vi "AnalogInput_PanelSim_Global.vi"(0 "menu":T5=enum."set avg_bits", 5 "Channel":T4, 9 "Value Set":dbl format="%#.4f", 11 "error in (no error)":errorcluster, 12 "String Value":string) -> (10 "AI Value out":T1={"type"="AI", "device"="", "name"="", "data"={"<init"=FALSE, "<avg_bits"=0, "<oversample_bits"=0, ">voltage"=0.0, " Accum Object"={"<init"=FALSE, ">value"=0.0, ">count"=0, "<center"=0, "<deadband"=0}}}, 15 "error out":errorcluster)   [LabVIEW 2019]
doc: "This is used to set and get the last motor output values. This is needed for simulation, since we cannot read these values from the hardware.\n\nThis software is licensed. Open the labview\\readme\\WPI Robotics Library Open Source License.txt file for more information."
uses:
  AI Accum proto.ctl
  AI Data proto.ctl
  AI proto.ctl
  <vilib>/Rock Robotics/SystemInterfaces/AI/FPGA_AIChannel.ctl
  AI Update Ops.ctl
panel:
  out "All Values":T1[](array[typedef])
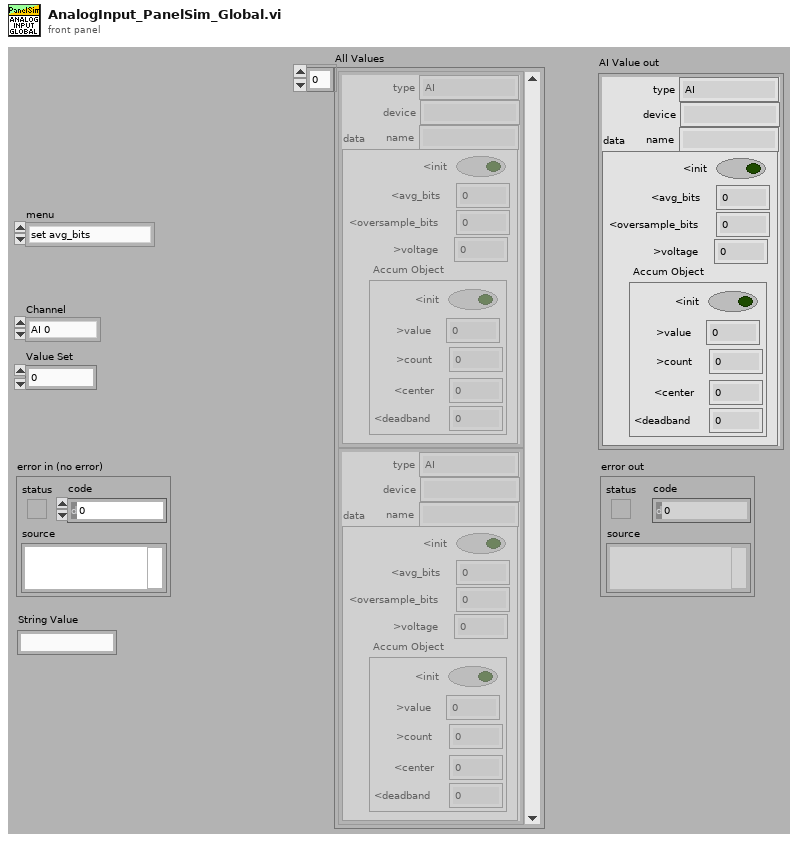
[diagram p1: front panel]
types:
  T1 = typedef "AI proto.ctl" = cluster{"type":string, "device":string, "name":string, "data":T2}
  T2 = typedef "AI Data proto.ctl" = cluster{"<init":bool, "<avg_bits":i32, "<oversample_bits":i32, ">voltage":dbl, " Accum Object":T3}
  T3 = typedef "AI Accum proto.ctl" = cluster{"<init":bool, ">value":dbl, ">count":i32, "<center":i32, "<deadband":i32}
  T4 = typedef "FPGA_AIChannel.ctl" = enum8{"AI 0", "AI 1", "AI 2", "AI 3", "AI MXP 0", "AI MXP 1", "AI MXP 2", "AI MXP 3", "Invalid"}
  T5 = typedef "AI Update Ops.ctl" = enum16{"set init", "set avg_bits", "set oversample_bits", "set voltage", "set Accum_init", "set Accum_value", "set Accum_count", "set Accum_center", "set Accum_deadband", "get", "delete", "JSON update", "set  name", "transmit initial", "reset"}
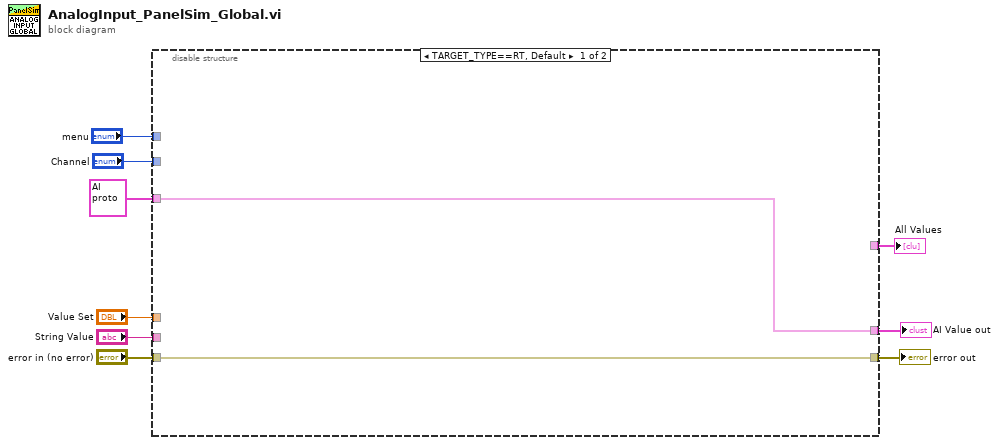
[diagram p0: block diagram]
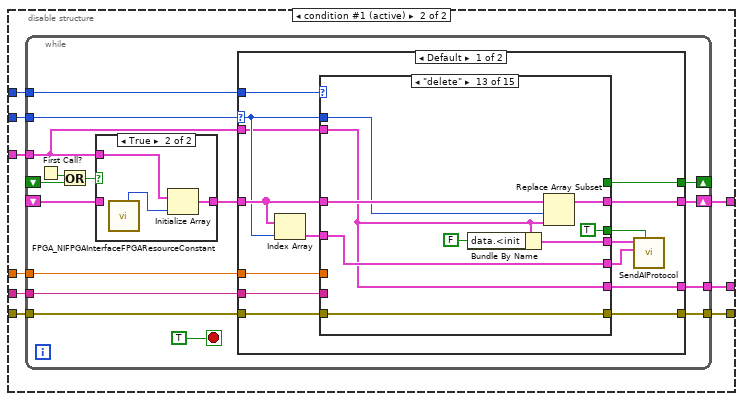
[diagram p2: hidden frame]
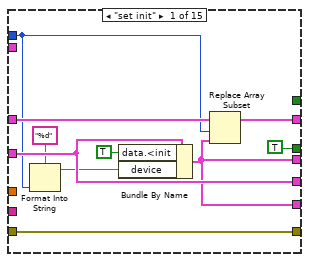
[diagram p3: hidden frame]
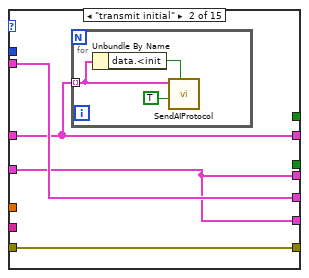
[diagram p4: hidden frame]
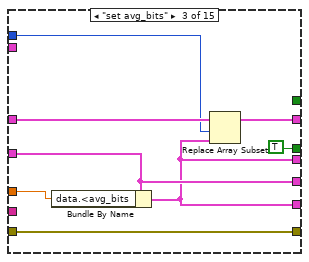
[diagram p5: hidden frame]
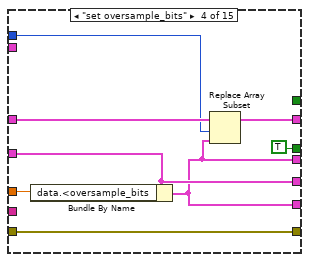
[diagram p6: hidden frame]
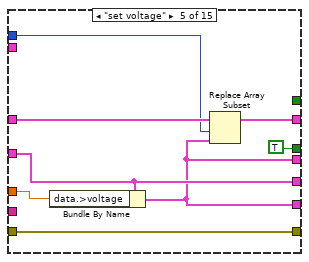
[diagram p7: hidden frame]
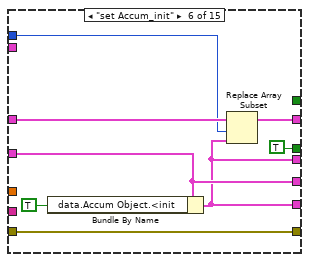
[diagram p8: hidden frame]
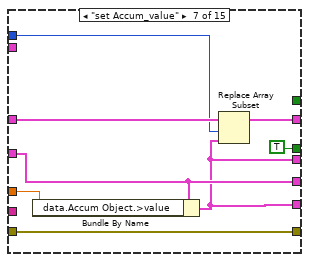
[diagram p9: hidden frame]
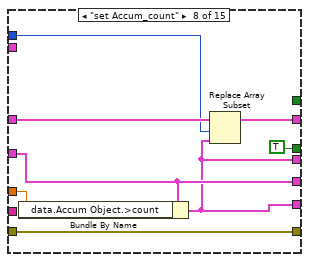
[diagram p10: hidden frame]
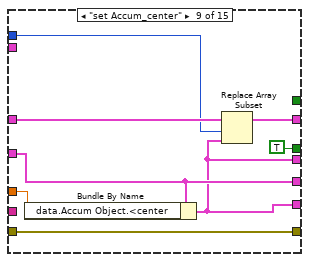
[diagram p11: hidden frame]
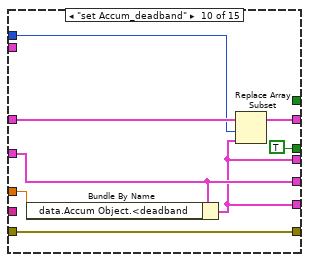
[diagram p12: hidden frame]
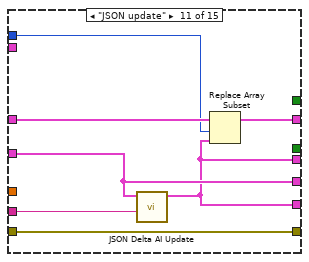
[diagram p13: hidden frame]
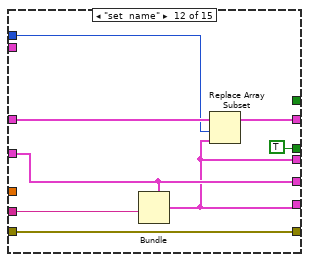
[diagram p14: hidden frame]
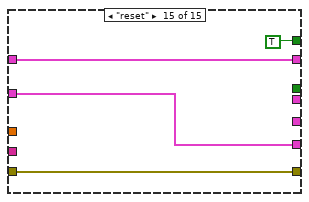
[diagram p16: hidden frame]
diagram:
  n1 = disable-structure shown="TARGET_TYPE==RT, Default" {
    disable-tunnel: "menu" -> [_ w20]
    disable-tunnel: [w11 w19] -> w8
    disable-tunnel: "error in (no error)" -> [w11 w18]
    disable-tunnel: [_ w17] -> w6
    disable-tunnel: "Value Set" -> [_ w16]
    disable-tunnel: "Channel" -> [_ w15]
    disable-tunnel: [w10 w14] -> w1
    disable-tunnel: T1 {"type"="AI", "device"="", "name"="", "data"={"<init"=FALSE, "<avg_bits"=0, "<oversample_bits"=0, ">voltage"=0.0, " Accum Object"={"<init"=FALSE, ">value"=0.0, ">count"=0, "<center"=0, "<deadband"=0}}} -> [w10 w13]
    disable-tunnel: "String Value" -> [_ w12]
    frame condition #0 {
    }
    frame condition #1 (active) {
      n2 = while {
        tunnel: w16 -> [w36]
        tunnel: w18 -> [w32]
        shift-right: [w35] -> w17
        shift-left: _ -> [w28]
        tunnel: [w34] -> w14
        tunnel: w20 -> [w33]
        tunnel: [w31] -> w19
        tunnel: w15 -> [w27]
        tunnel: w13 -> [w26]
        tunnel: w12 -> [w25]
        shift-right: [w21] -> _
        shift-left: _ -> [w22]
        stop <- TRUE stop-if-true
        n3 = First Call?() -> (First Call?: T/F=w23:bool)
        n4 = Or(x=w23, y=w22) -> (x .or. y?=w24:bool)
        n5 = case shown="True" w24 {
          tunnel: [w167 w170] -> w29
          tunnel: w28 -> [w167 _]
          tunnel: w26 -> [_ w169]
          frame False {
          }
          frame True {
            n6 = call <vilib>:"FPGA_NIFPGAInterfaceFPGAResourceConstant.vi"() -> ("NumberOfAIChannels"=w168:u8)  [unwired: 11 out]
            n7 = Initialize Array(w169, w168) -> (w170:T1[])
          }
        }
        n8 = case shown="Default" w27 {
          selector: w27 -> [w44 _]
          tunnel: w36 -> [w51 _]
          tunnel: [w50 w166] -> w35
          tunnel: [w49 w164] -> w34
          tunnel: w33 -> [w48 _]
          tunnel: w32 -> [w47 w165]
          tunnel: [w46 w165] -> w31
          tunnel: w29 -> [w45 w166]
          tunnel: w26 -> [w42 w164]
          tunnel: w25 -> [w38 _]
          tunnel: [w37 _] -> w21
          frame Default {
            n9 = Index Array(array=w45, index=w44) -> (element=w43:T1)
            n10 = case shown="\"delete\"" w48 {
              tunnel: w51 -> [_ _ w71 w78 w86 _ w103 w111 w119 w126 _ _ _ _ _]
              tunnel: [w61 w62 w76 w84 w92 w100 w108 w116 w124 w132 w139 w147 w155 w159 w163] -> w50
              tunnel: w45 -> [w59 w62 w74 w82 w90 w98 w106 w114 w122 w130 w137 w145 w156 w159 w163]
              tunnel: [w55 w63 w69 w77 w85 w93 w101 w109 w117 w125 w133 w140 w149 w157 w161] -> w49
              tunnel: [w60 w65 w75 w83 w91 w99 w107 w115 w123 w131 w138 w146 w154 w158 w162] -> w46
              tunnel: w47 -> [w60 w65 w75 w83 w91 w99 w107 w115 w123 w131 w138 w146 w154 w158 w162]
              tunnel: w44 -> [w54 _ w72 w80 w88 w96 w104 w112 w120 w128 w136 w143 w151 _ _]
              tunnel: [w55 w63 w69 w77 w85 w93 w101 w109 w117 w125 w133 w140 w150 _ _] -> w41
              tunnel: [w57 w64 w70 w79 w87 w94 w102 w110 w118 w127 w134 w142 w152 _ _] -> w40
              tunnel: [TRUE _ TRUE TRUE TRUE TRUE TRUE TRUE TRUE TRUE _ TRUE TRUE _ _] -> w39
              tunnel: w43 -> [w57 w63 w70 w79 w87 w94 w102 w110 w118 w127 w134 w142 w152 w157 w161]
              tunnel: w42 -> [_ w64 _ _ _ _ _ _ _ _ _ _ w149 _ _]
              tunnel: w38 -> [_ _ _ _ _ _ _ _ _ _ w135 w141 _ _ _]
              tunnel: [_ _ _ _ _ _ _ _ _ _ _ _ _ _ TRUE] -> w37
              frame "set init" {
                n11 = Format Into String(format string="%d", w54) -> (resulting string=w53:string)  [unwired: 2 in, 1 out]
                n12 = Bundle By Name(cluster=w57, "data.<init"=TRUE, "device"=w53) -> (w55:T1)
                n13 = Replace Array Subset(array=w59, new element=w55, index=w54) -> (w61:T1[])
              }
              frame "transmit initial" {
                n14 = for {
                  tunnel: w62 -> [w67] mode=indexing
                  n15 = Unbundle By Name(w67) -> ("data.<init"=w66:bool)
                  n16 = call "SendAIProtocol.vi"("Send"=w66, "Initialize"=TRUE ("Send"), "AI new"=w67) -> ()  [unwired: 9 in]
                }
              }
              frame "set avg_bits" {
                n17 = Bundle By Name(cluster=w70, "data.<avg_bits"=w71) -> (w69:T1)
                n18 = Replace Array Subset(array=w74, new element=w69, index=w72) -> (w76:T1[])
              }
              frame "set oversample_bits" {
                n19 = Bundle By Name(cluster=w79, "data.<oversample_bits"=w78) -> (w77:T1)
                n20 = Replace Array Subset(array=w82, new element=w77, index=w80) -> (w84:T1[])
              }
              frame "set voltage" {
                n21 = Bundle By Name(cluster=w87, "data.>voltage"=w86) -> (w85:T1)
                n22 = Replace Array Subset(array=w90, new element=w85, index=w88) -> (w92:T1[])
              }
              frame "set Accum_init" {
                n23 = Bundle By Name(cluster=w94, "data.Accum Object.<init"=TRUE) -> (w93:T1)
                n24 = Replace Array Subset(array=w98, new element=w93, index=w96) -> (w100:T1[])
              }
              frame "set Accum_value" {
                n25 = Bundle By Name(cluster=w102, "data.Accum Object.>value"=w103) -> (w101:T1)
                n26 = Replace Array Subset(array=w106, new element=w101, index=w104) -> (w108:T1[])
              }
              frame "set Accum_count" {
                n27 = Bundle By Name(cluster=w110, "data.Accum Object.>count"=w111) -> (w109:T1)
                n28 = Replace Array Subset(array=w114, new element=w109, index=w112) -> (w116:T1[])
              }
              frame "set Accum_center" {
                n29 = Bundle By Name(cluster=w118, "data.Accum Object.<center"=w119) -> (w117:T1)
                n30 = Replace Array Subset(array=w122, new element=w117, index=w120) -> (w124:T1[])
              }
              frame "set Accum_deadband" {
                n31 = Bundle By Name(cluster=w127, "data.Accum Object.<deadband"=w126) -> (w125:T1)
                n32 = Replace Array Subset(array=w130, new element=w125, index=w128) -> (w132:T1[])
              }
              frame "JSON update" {
                n33 = call "JSON Delta AI Update.vi"("Delta JSON"=w135, "input"=w134) -> ("output"=w133:T1)  [unwired: 8 in, 1 out]
                n34 = Replace Array Subset(array=w137, new element=w133, index=w136) -> (w139:T1[])
              }
              frame "set  name" {
                n35 = Bundle(cluster=w142, "name"=w141) -> (w140:T1)  [unwired: 3 in]
                n36 = Replace Array Subset(array=w145, new element=w140, index=w143) -> (w147:T1[])
              }
              frame "delete" {
                n37 = Bundle By Name(cluster=w149, "data.<init"=FALSE) -> (w150:T1)
                n38 = Replace Array Subset(array=w156, new element=w149, index=w151) -> (w155:T1[])
              }
              frame "get" {
              }
              frame "reset" {
              }
            }
            n39 = call "SendAIProtocol.vi"("Send"=w39, "AI prev"=w40, "AI new"=w41) -> ()  [unwired: 9 in]
          }
          frame "Invalid" {
            # "Do nothing if \nchannel is Invalid."
          }
        }
      }
    }
  }
  "error out" <- w8
  "AI Value out" <- w1
  "All Values" <- w6
